vi "Actor Core.vi"(8 "error in":errorcluster, 11 "Simple Actor in":refnum<class "Simple Actor.lvclass">) -> (0 "error out":errorcluster, 3 "Actor out":refnum<class "Actor.lvclass">)   [LabVIEW 2012, in "Simple Actor.lvclass"]
doc: "Receives messages to the actor, reacts to them, and initiates any error handling that may shut the actor down.\n\nDescendant classes can override this VI to append parallel tasks for the actor to complete while it handles messages. Overrides must use the Call Parent Method node."
uses:
  Simple Actor.lvclass
  <vilib>/ActorFramework/Actor/Actor.lvclass
  Simple Actor.lvclass/Simple Actor.ctl
  <vilib>/ActorFramework/Actor/Actor.lvclass/Actor.ctl
  <vilib>/ActorFramework/Message Enqueuer/Message Enqueuer.lvclass/Message Enqueuer.ctl
  <vilib>/ActorFramework/Message Enqueuer/Init from Existing Queue.vi
  <vilib>/ActorFramework/Message Enqueuer/Enqueue.vi
  <vilib>/ActorFramework/Message Priority Queue/Priority Enqueue.vi
  <vilib>/ActorFramework/Message Enqueuer/Message Enqueuer.lvclass
  Simple Actor Messages/Update Msg/Update Msg.lvclass
panel:
  out "Stop":bool
  out "Gauge":dbl(knob) scale=0.0..10.0
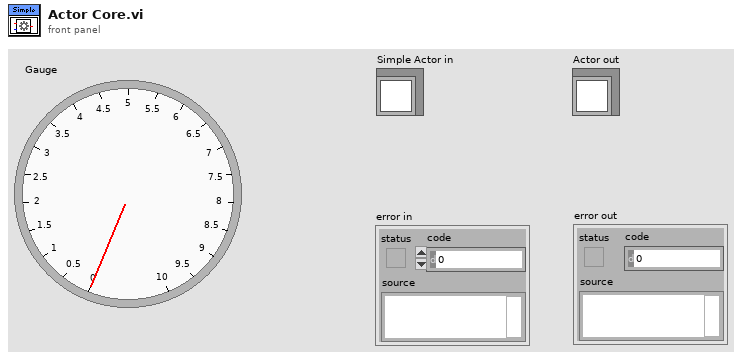
[diagram p1: front panel]
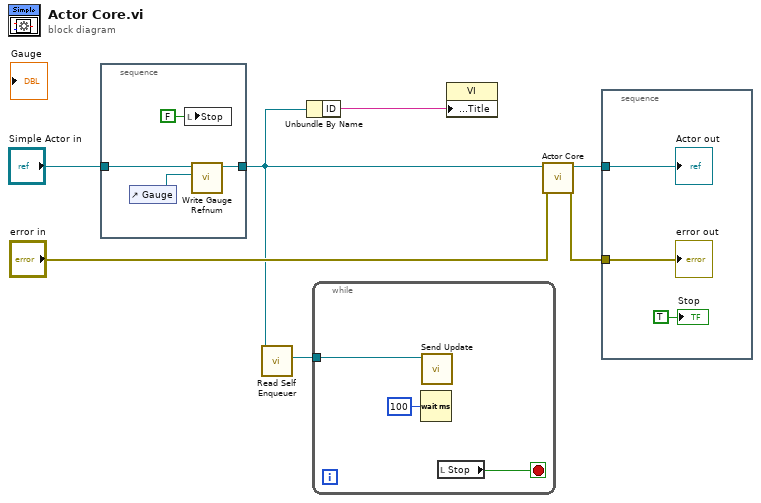
[diagram p0: block diagram]
diagram:
  n1 = stacked-sequence {
    tunnel: "Simple Actor in" -> [w11]
    tunnel: [w9] -> w2
    frame #0 {
      n2 = control-ref of="Gauge"() -> (w10:refnum<vi>)
      n3 = local write "Stop"(FALSE ("Stop")) -> ()
      n4 = call "Write Gauge Refnum.vi"("Gauge Refnum"=w10, "Simple Actor in"=w11) -> ("Simple Actor out"=w9:refnum<class "Simple Actor.lvclass">)  [unwired: 9 in]
    }
  }
  n5 = call <vilib>:"Read Self Enqueuer.vi"("Actor"=w2) -> ("Self Enqueuer"=w3:refnum<class "Message Enqueuer.lvclass">)  [unwired: 10 in]
  n6 = Unbundle By Name(w2) -> ("ID"=w1:string)
  n7 = while {
    tunnel: w3 -> [w14]
    stop <- w13 stop-if-true
    n8 = Wait (ms)(milliseconds to wait=u32 100) -> ()  [unwired: 1 out]
    n9 = call "Send Update.vi"("Message Enqueuer"=w14) -> ()  [unwired: 9 in, 2 out]
    n10 = local read "Stop"() -> (w13:bool)
  }
  n11 = property class="VI"("Front Panel.Title"=w1) -> ()  [unwired: 2 in, 2 out]
  n12 = call-parent "Actor Core.vi"("error in"="error in", "Actor in"=w2) -> ("error out"=w5:errorcluster, "Actor out"=w7:refnum<class "Actor.lvclass">)  [unwired: 8 in]
  n13 = stacked-sequence {
    tunnel: w7 -> [w17]
    tunnel: w5 -> [w16]
    frame #0 {
      "error out" <- w16
      "Actor out" <- w17
      "Stop" <- TRUE ("Stop")
    }
  }
